vi "Encode boolean.vi"(8 "error in (no error)":errorcluster, 11 "Data":variant) -> (0 "error out":errorcluster, 3 "String":string)   [LabVIEW 2026, in "TALOS.lvlib" / "Guardian.lvlib" / "Guardian.lvclass"]
uses:
  Guardian.lvclass
  TALOS.lvlib
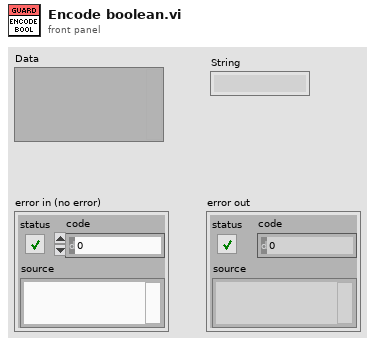
[diagram p1: front panel]
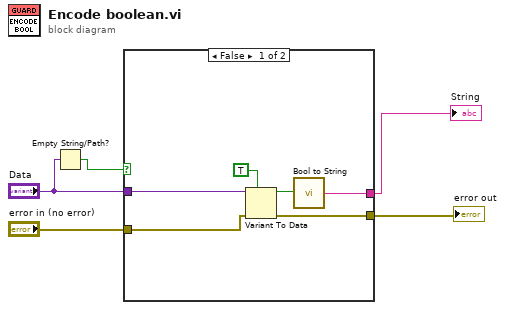
[diagram p0: block diagram]
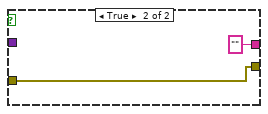
[diagram p2: hidden frame]
diagram:
  n1 = Empty String/Path?(string/path="Data") -> (empty?=w1:bool)
  n2 = case shown="False" w1 {
    tunnel: [w11 w12] -> w5
    tunnel: [w10 "" ("String")] -> w4
    tunnel: "error in (no error)" -> [w7 w12]
    tunnel: "Data" -> [w6 _]
    frame False {
      n3 = Variant To Data(error in=w7, type=TRUE ("Local also?"), Variant=w6) -> (data=w9:bool, error out=w11:errorcluster)
      n4 = call "Bool to String.vi"("Boolean"=w9) -> ("String"=w10:string)
    }
    frame True {
    }
  }
  "error out" <- w5
  "String" <- w4
